vi "Database.Handler.GetDBtime.vi"(8 "error in (no error)":errorcluster, 11 "Data in":T1) -> (0 "error out":errorcluster, 3 "Data out":T1)   [LabVIEW 2016]
doc: "Get database time\n\nWabco 2017 All right reserved\nAuthor: maciej.szupienko@wabco-auto.com"
uses:
  Database.Handler.Data.ctl
  Database.Handler.Data.Status.ctl
  Database.Handler.Data.Sets.ctl
  Tools/EventLog/EventLog.EventSource.ctl
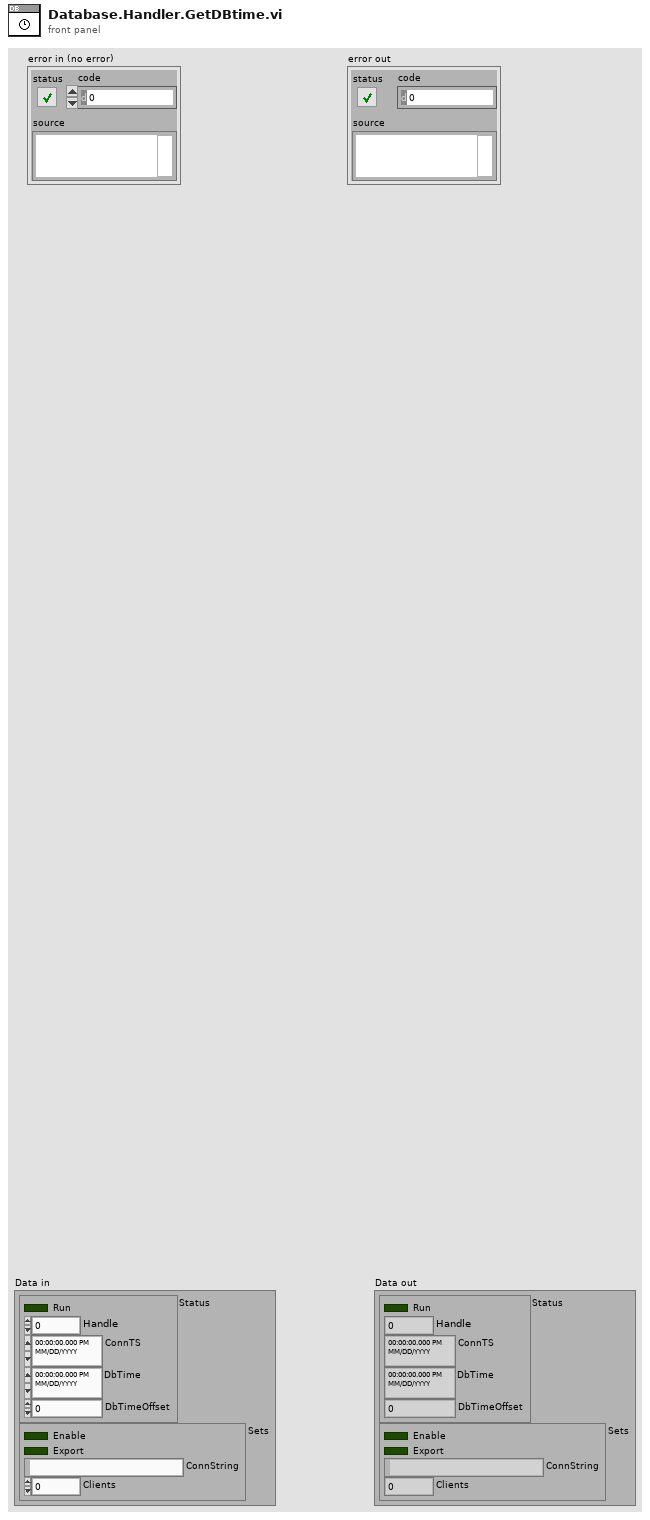
[diagram p1: front panel]
types:
  T1 = typedef "Database.Handler.Data.ctl" = cluster{"Status":T2, "Sets":T3}
  T2 = typedef "Database.Handler.Data.Status.ctl" = cluster{"Run":bool, "Handle":i32, "ConnTS":timestamp, "DbTime":timestamp, "DbTimeOffset":dbl}
  T3 = typedef "Database.Handler.Data.Sets.ctl" = cluster{"Enable":bool, "Export":bool, "ConnString":string, "Clients":i32}
  T4 = typedef "EventLog.EventSource.ctl" = enum16{"All", "Gui", "Cache", "PLC1", "PLC2", "PLC3", "DB", "DB01", "DB02", "DB03", "DB04", "DB05", "DB06", "DB07", "DB08", "DB09", "DB10", "DB11", "DB12", "DB13", "DB14", "DB15", "DB16"}
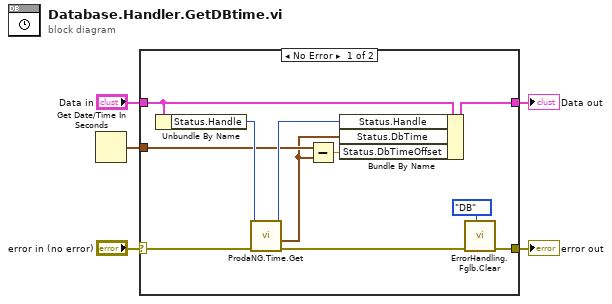
[diagram p0: block diagram]
diagram:
  n1 = Get Date/Time In Seconds() -> (seconds since 1Jan1904=w1:timestamp)
  n2 = case shown="No Error" "error in (no error)" {
    selector: "error in (no error)" -> [w15 w18]
    tunnel: [w10 w18] -> w2
    tunnel: [w12 w17] -> w5
    tunnel: "Data in" -> [w13 w17]
    tunnel: w1 -> [w9 _]
    frame No Error {
      n3 = Unbundle By Name(w13) -> ("Status.Handle"=w14:i32)
      n4 = call "ProdaNG.Time.Get.vi"("error in"=w15, "dbHandleIn"=w14) -> ("error out"=w11:errorcluster, "time"=w8:timestamp, "dbHandle"=w16:i32)  [unwired: 5 in, 1 out]
      n5 = Subtract(x=w9, y=w8) -> (x-y=w7:dbl)
      n6 = Bundle By Name(cluster=w13, "Status.Handle"=w16, "Status.DbTime"=w8, "Status.DbTimeOffset"=w7) -> (w12:T1)
      n7 = call "ErrorHandling.Fglb.Clear.vi"("Event source"=EventLog.EventSource."DB", "error in (no error)"=w11) -> ("error out"=w10:errorcluster)  [unwired: 9 in]
    }
    frame Error {
    }
  }
  "error out" <- w2
  "Data out" <- w5
